vi "TekDrive Upload Example.vi"() -> ()   [LabVIEW 2018]
panel:
  in  "file":path
  in  "Access Key":string="OcLByW5QBVjdY2iTYvcr06MEpdy9pgQxtqk5VFBVCMe3BDEm"
  in  "Parent Folder ID (optional)":string="ec812d06-2310-4cc5-9075-4b74d782c211"
  out "error out":errorcluster
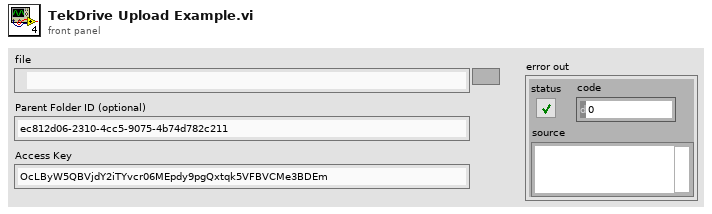
[diagram p1: front panel]
types:
  T1 = typedef "TekDriveSession.ctl" = cluster{"Access Key":string, "HTTP Client Handle":T2}
  T2 = typedef "LabVIEWHTTPClient.lvlib/ClientHandle.ctl" = refnum<k1>
  T3 = typedef "File Model.ctl" = cluster{"id":string, "parentFolderId":string, "owner":cluster{"id":string, "username":string}, "creator":cluster{"id":string, "username":string}, "name":string, "type":string, "fileType":string, "uploadState":string, "createdAt":string, "updatedAt":string, "sharedAt":string, "bytes":string, "permissions":cluster{"owner":bool, "creator":bool, "read":bool, "edit":bool, "public":bool}}
  T4 = cluster{"file":T3, "uploadUrl":string, "storageLimitExceeded":bool}
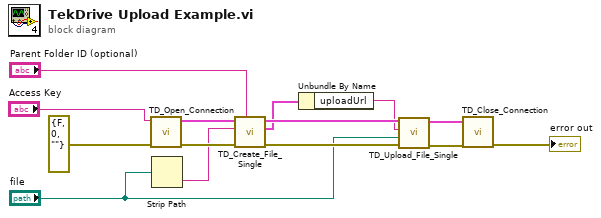
[diagram p0: block diagram]
diagram:
  n1 = call "TD_Open_Connection.vi"("Error In"=errorcluster {"status"=FALSE, "code"=0, "source"=""}, "Access Key"="Access Key") -> ("Error Out"=w11:errorcluster, "TekDrive Session"=w12:T1)  [unwired: 8 in]
  n2 = Strip Path(path="file") -> (name=w1:string)  [unwired: 1 out]
  n3 = call "TD_Create_File_Single.vi"("Parent Folder ID (optional)"="Parent Folder ID (optional)", "error in (no error)"=w11, "File name"=w1, "TekDrive Session"=w12) -> ("error out"=w6:errorcluster, "value"=w4:T4, "TekDrive Session 2"=w5:T1)  [unwired: 3 in, 2 out]
  n4 = Unbundle By Name(w4) -> ("uploadUrl"=w3:string)
  n5 = call "TD_Upload_File_Single.vi"("error in (no error)"=w6, "file"="file", "Upload Url"=w3, "TekDrive Session In"=w5) -> ("error out"=w7:errorcluster, "TekDrive Session Out"=w8:T1)  [unwired: 6 in]
  n6 = call "TD_Close_Connection.vi"("error in (no error)"=w7, "TekDrive Session"=w8) -> ("error out"=→"error out":errorcluster)  [unwired: 9 in]
